vi "read Txt Files.vi"(10 "file path (use dialog)":path) -> (1 "error out":errorcluster, 2 "number":T1)   [LabVIEW 2017] (continued)
0.000000\tVoltage¡G\t-0.001160\nReal Periold(ms)¡G\t1\tEncoder Position(0.1mm)¡G\t0.000000\tVelocity(0.1mm0/s)¡G\t0.000000\tVoltage¡G\t0.000732\nReal Periold(ms)¡G\t1\tEncoder Position(0.1mm)¡G\t0.000000\tVelocity(0.1mm0/s)¡G\t0.000000\tVoltage¡G\t-0.003082\nReal Periold(ms)¡G\t1\tEncoder Position(0.1mm)¡G\t0.000000\tVelocity(0.1mm0/s)¡G\t0.000000\tVoltage¡G\t0.002319\nReal Periold(ms)¡G\t1\tEncoder Position(0.1mm)¡G\t0.000000\tVelocity(0.1mm0/s)¡G\t0.000000\tVoltage¡G\t-0.005310\nReal Periold(ms)¡G\t1\tEncoder Position(0.1mm)¡G\t0.000000\tVelocity(0.1mm0/s)¡G\t0.000000\tVoltage¡G\t-0.011688\nReal Periold(ms)¡G\t1\tEncoder Position(0.1mm)¡G\t0.000000\tVelocity(0.1mm0/s)¡G\t0.000000\tVoltage¡G\t-0.005005\nReal Periold(ms)¡G\t1\tEncoder Position(0.1mm)¡G\t0.000000\tVelocity(0.1mm0/s)¡G\t0.000000\tVoltage¡G\t0.002319\nReal Periold(ms)¡G\t1\tEncoder Position(0.1mm)¡G\t0.000000\tVelocity(0.1mm0/s)¡G\t0.000000\tVoltage¡G\t-0.006256\nReal Periold(ms)¡G\t1\tEncoder Position(0.1mm)¡G\t0.000000\tVelocity(0.1mm0/s)¡G\t0.000000\tVoltage¡G\t0.007751\nReal Periold(ms)¡G\t1\tEncoder Position(0.1mm)¡G\t0.000000\tVelocity(0.1mm0/s)¡G\t0.000000\tVoltage¡G\t0.001678\nReal Periold(ms)¡G\t1\tEncoder Position(0.1mm)¡G\t0.000000\tVelocity(0.1mm0/s)¡G\t0.000000\tVoltage¡G\t-0.000214\nReal Periold(ms)¡G\t1\tEncoder Position(0.1mm)¡G\t0.000000\tVelocity(0.1mm0/s)¡G\t0.000000\tVoltage¡G\t-0.006592\nReal Periold(ms)¡G\t1\tEncoder Position(0.1mm)¡G\t0.000000\tVelocity(0.1mm0/s)¡G\t0.000000\tVoltage¡G\t0.003296\nReal Periold(ms)¡G\t1\tEncoder Position(0.1mm)¡G\t0.000000\tVelocity(0.1mm0/s)¡G\t0.000000\tVoltage¡G\t0.005188\nReal Periold(ms)¡G\t1\tEncoder Position(0.1mm)¡G\t0.000000\tVelocity(0.1mm0/s)¡G\t0.000000\tVoltage¡G\t0.007111\nReal Periold(ms)¡G\t1\tEncoder Position(0.1mm)¡G\t0.000000\tVelocity(0.1mm0/s)¡G\t0.000000\tVoltage¡G\t-0.003387\nReal Periold(ms)¡G\t1\tEncoder Position(0.1mm)¡G\t0.000000\tVelocity(0.1mm0/s)¡G\t0.000000\tVoltage¡G\t0.001068\nReal Periold(ms)¡G\t1\tEncoder Position(0.1mm)¡G\t0.000000\tVelocity(0.1mm0/s)¡G\t0.000000\tVoltage¡G\t-0.004364\nReal Periold(ms)¡G\t1\tEncoder Position(0.1mm)¡G\t0.000000\tVelocity(0.1mm0/s)¡G\t0.000000\tVoltage¡G\t-0.001160\nReal Periold(ms)¡G\t1\tEncoder Position(0.1mm)¡G\t0.000000\tVelocity(0.1mm0/s)¡G\t0.000000\tVoltage¡G\t0.001068\nReal Periold(ms)¡G\t1\tEncoder Position(0.1mm)¡G\t0.000000\tVelocity(0.1mm0/s)¡G\t0.000000\tVoltage¡G\t0.006775\nReal Periold(ms)¡G\t1\tEncoder Position(0.1mm)¡G\t0.000000\tVelocity(0.1mm0/s)¡G\t0.000000\tVoltage¡G\t0.001373\nReal Periold(ms)¡G\t1\tEncoder Position(0.1mm)¡G\t0.000000\tVelocity(0.1mm0/s)¡G\t0.000000\tVoltage¡G\t-0.005615\nReal Periold(ms)¡G\t1\tEncoder Position(0.1mm)¡G\t0.000000\tVelocity(0.1mm0/s)¡G\t0.000000\tVoltage¡G\t-0.003723\nReal Periold(ms)¡G\t1\tEncoder Position(0.1mm)¡G\t0.000000\tVelocity(0.1mm0/s)¡G\t0.000000\tVoltage¡G\t0.003601\nReal Periold(ms)¡G\t1\tEncoder Position(0.1mm)¡G\t0.000000\tVelocity(0.1mm0/s)¡G\t0.000000\tVoltage¡G\t0.063446\nReal Periold(ms)¡G\t1\tEncoder Position(0.1mm)¡G\t0.000000\tVelocity(0.1mm0/s)¡G\t0.000000\tVoltage¡G\t-0.000214\nReal Periold(ms)¡G\t1\tEncoder Position(0.1mm)¡G\t0.000000\tVelocity(0.1mm0/s)¡G\t0.000000\tVoltage¡G\t0.006775\nReal Periold(ms)¡G\t1\tEncoder Position(0.1mm)¡G\t0.000000\tVelocity(0.1mm0/s)¡G\t0.000000\tVoltage¡G\t0.002655\nReal Periold(ms)¡G\t1\tEncoder Position(0.1mm)¡G\t0.000000\tVelocity(0.1mm0/s)¡G\t0.000000\tVoltage¡G\t-0.016754\nReal Periold(ms)¡G\t1\tEncoder Position(0.1mm)¡G\t0.000000\tVelocity(0.1mm0/s)¡G\t0.000000\tVoltage¡G\t0.001373\nReal Periold(ms)¡G\t1\tEncoder Position(0.1mm)¡G\t0.000000\tVelocity(0.1mm0/s)¡G\t0.000000\tVoltage¡G\t-0.005310\nReal Periold(ms)¡G\t1\tEncoder Position(0.1mm)¡G\t0.000000\tVelocity(0.1mm0/s)¡G\t0.000000\tVoltage¡G\t0.005188\nReal Periold(ms)¡G\t1\tEncoder Position(0.1mm)¡G\t0.000000\tVelocity(0.1mm0/s)¡G\t0.000000\tVoltage¡G\t-0.005005\nReal Periold(ms)¡G\t1\tEncoder Position(0.1mm)¡G\t0.000000\tVelocity(0.1mm0/s)¡G\t0.000000\tVoltage¡G\t0.013794\nReal Periold(ms)¡G\t1\tEncoder Position(0.1mm)¡G\t0.000000\tVelocity(0.1mm0/s)¡G\t0.000000\tVoltage¡G\t0.003906\nReal Periold(ms)¡G\t1\tEncoder Position(0.1mm)¡G\t0.000000\tVelocity(0.1mm0/s)¡G\t0.000000\tVoltage¡G\t0.052307\nReal Periold(ms)¡G\t1\tEncoder Position(0.1mm)¡G\t0.000000\tVelocity(0.1mm0/s)¡G\t0.000000\tVoltage¡G\t-0.006897\nReal Periold(ms)¡G\t1\tEncoder Position(0.1mm)¡G\t0.000000\tVelocity(0.1mm0/s)¡G\t0.000000\tVoltage¡G\t-0.028229\nReal Periold(ms)¡G\t1\tEncoder Position(0.1mm)¡G\t0.000000\tVelocity(0.1mm0/s)¡G\t0.000000\tVoltage¡G\t-0.000214\nReal Periold(ms)¡G\t1\tEncoder Position(0.1mm)¡G\t0.000000\tVelocity(0.1mm0/s)¡G\t0.000000\tVoltage¡G\t-0.008179\nReal Periold(ms)¡G\t1\tEncoder Position(0.1mm)¡G\t0.000000\tVelocity(0.1mm0/s)¡G\t0.000000\tVoltage¡G\t0.000732\nReal Periold(ms)¡G\t1\tEncoder Position(0.1mm)¡G\t0.000000\tVelocity(0.1mm0/s)¡G\t0.000000\tVoltage¡G\t-0.017395\nReal Periold(ms)¡G\t1\tEncoder Position(0.1mm)¡G\t0.000000\tVelocity(0.1mm0/s)¡G\t0.000000\tVoltage¡G\t-0.005615\nReal Periold(ms)¡G\t1\tEncoder Position(0.1mm)¡G\t0.000000\tVelocity(0.1mm0/s)¡G\t0.000000\tVoltage¡G\t-0.001495\nReal Periold(ms)¡G\t1\tEncoder Position(0.1mm)¡G\t0.000000\tVelocity(0.1mm0/s)¡G\t0.000000\tVoltage¡G\t0.001678\nReal Periold(ms)¡G\t1\tEncoder Position(0.1mm)¡G\t0.000000\tVelocity(0.1mm0/s)¡G\t0.000000\tVoltage¡G\t0.002655\nReal Periold(ms)¡G\t1\tEncoder Position(0.1mm)¡G\t0.000000\tVelocity(0.1mm0/s)¡G\t0.000000\tVoltage¡G\t0.000092\nReal Periold(ms)¡G\t1\tEncoder Position(0.1mm)¡G\t0.000000\tVelocity(0.1mm0/s)¡G\t0.000000\tVoltage¡G\t-0.046997\nReal Periold(ms)¡G\t1\tEncoder Position(0.1mm)¡G\t0.000000\tVelocity(0.1mm0/s)¡G\t0.000000\tVoltage¡G\t-0.008820\nReal Periold(ms)¡G\t1\tEncoder Position(0.1mm)¡G\t0.000000\tVelocity(0.1mm0/s)¡G\t0.000000\tVoltage¡G\t0.010284\nReal Periold(ms)¡G\t1\tEncoder Position(0.1mm)¡G\t0.000000\tVelocity(0.1mm0/s)¡G\t0.000000\tVoltage¡G\t0.009003\nReal Periold(ms)¡G\t1\tEncoder Position(0.1mm)¡G\t0.000000\tVelocity(0.1mm0/s)¡G\t0.000000\tVoltage¡G\t-0.008820\nReal Periold(ms)¡G\t1\tEncoder Position(0.1mm)¡G\t0.000000\tVelocity(0.1mm0/s)¡G\t0.000000\tVoltage¡G\t0.000427\nReal Periold(ms)¡G\t1\tEncoder Position(0.1mm)¡G\t0.000000\tVelocity(0.1mm0/s)¡G\t0.000000\tVoltage¡G\t0.001068\nReal Periold(ms)¡G\t1\tEncoder Position(0.1mm)¡G\t0.000000\tVelocity(0.1mm0/s)¡G\t0.000000\tVoltage¡G\t-0.000214\nReal Periold(ms)¡G\t1\tEncoder Position(0.1mm)¡G\t0.000000\tVelocity(0.1mm0/s)¡G\t0.000000\tVoltage¡G\t-0.003387\nReal Periold(ms)¡G\t1\tEncoder Position(0.1mm)¡G\t0.000000\tVelocity(0.1mm0/s)¡G\t0.000000\tVoltage¡G\t-0.004669\nReal Periold(ms)¡G\t1\tEncoder Position(0.1mm)¡G\t0.000000\tVelocity(0.1mm0/s)¡G\t0.000000\tVoltage¡G\t0.005188\nReal Periold(ms)¡G\t1\tEncoder Position(0.1mm)¡G\t0.000000\tVelocity(0.1mm0/s)¡G\t0.000000\tVoltage¡G\t-0.005005\nReal Periold(ms)¡G\t1\tEncoder Position(0.1mm)¡G\t0.000000\tVelocity(0.1mm0/s)¡G\t0.000000\tVoltage¡G\t0.003296\nReal Periold(ms)¡G\t1\tEncoder Position(0.1mm)¡G\t0.000000\tVelocity(0.1mm0/s)¡G\t0.000000\tVoltage¡G\t0.002655\nReal Periold(ms)¡G\t1\tEncoder Position(0.1mm)¡G\t0.000000\tVelocity(0.1mm0/s)¡G\t0.000000\tVoltage¡G\t0.001678\nReal Periold(ms)¡G\t1\tEncoder Position(0.1mm)¡G\t0.000000\tVelocity(0.1mm0/s)¡G\t0.000000\tVoltage¡G\t-0.004028\nReal Periold(ms)¡G\t1\tEncoder Position(0.1mm)¡G\t0.000000\tVelocity(0.1mm0/s)¡G\t0.000000\tVoltage¡G\t0.002960\nReal Periold(ms)¡G\t1\tEncoder Position(0.1mm)¡G\t0.000000\tVelocity(0.1mm0/s)¡G\t0.000000\tVoltage¡G\t0.018250\nReal Periold(ms)¡G\t1\tEncoder Position(0.1mm)¡G\t0.000000\tVelocity(0.1mm0/s)¡G\t0.000000\tVoltage¡G\t0.007751\nReal Periold(ms)¡G\t1\tEncoder Position(0.1mm)¡G\t0.000000\tVelocity(0.1mm0/s)¡G\t0.000000\tVoltage¡G\t0.008698\nReal Periold(ms)¡G\t1\tEncoder Position(0.1mm)¡G\t0.000000\tVelocity(0.1mm0/s)¡G\t0.000000\tVoltage¡G\t-0.002441\nReal Periold(ms)¡G\t1\tEncoder Position(0.1mm)¡G\t0.000000\tVelocity(0.1mm0/s)¡G\t0.000000\tVoltage¡G\t-0.009460\nReal Periold(ms)¡G\t1\tEncoder Position(0.1mm)¡G\t0.000000\tVelocity(0.1mm0/s)¡G\t0.000000\tVoltage¡G\t-0.005310\nReal Periold(ms)¡G\t1\tEncoder Position(0.1mm)¡G\t0.000000\tVelocity(0.1mm0/s)¡G\t0.000000\tVoltage¡G\t-0.000549\nReal Periold(ms)¡G\t1\tEncoder Position(0.1mm)¡G\t0.000000\tVelocity(0.1mm0/s)¡G\t0.000000\tVoltage¡G\t0.002319\nReal Periold(ms)¡G\t1\tEncoder Position(0.1mm)¡G\t0.000000\tVelocity(0.1mm0/s)¡G\t0.000000\tVoltage¡G\t-0.014526\nReal Periold(ms)¡G\t1\tEncoder Position(0.1mm)¡G\t0.000000\tVelocity(0.1mm0/s)¡G\t0.000000\tVoltage¡G\t-0.012939\nReal Periold(ms)¡G\t1\tEncoder Position(0.1mm)¡G\t0.000000\tVelocity(0.1mm0/s)¡G\t0.000000\tVoltage¡G\t0.006470\nReal Periold(ms)¡G\t1\tEncoder Position(0.1mm)¡G\t0.000000\tVelocity(0.1mm0/s)¡G\t0.000000\tVoltage¡G\t0.001068\nReal Periold(ms)¡G\t1\tEncoder Position(0.1mm)¡G\t0.000000\tVelocity(0.1mm0/s)¡G\t0.000000\tVoltage¡G\t-0.003387\nReal Periold(ms)¡G\t1\tEncoder Position(0.1mm)¡G\t0.000000\tVelocity(0.1mm0/s)¡G\t0.000000\tVoltage¡G\t0.008057\nReal Periold(ms)¡G\t1\tEncoder Position(0.1mm)¡G\t0.000000\tVelocity(0.1mm0/s)¡G\t0.000000\tVoltage¡G\t-0.001801\nReal Periold(ms)¡G\t1\tEncoder Position(0.1mm)¡G\t0.000000\tVelocity(0.1mm0/s)¡G\t0.000000\tVoltage¡G\t0.003296\nReal Periold(ms)¡G\t1\tEncoder Position(0.1mm)¡G\t0.000000\tVelocity(0.1mm0/s)¡G\t0.000000\tVoltage¡G\t-0.007538\nReal Periold(ms)¡G\t1\tEncoder Position(0.1mm)¡G\t0.000000\tVelocity(0.1mm0/s)¡G\t0.000000\tVoltage¡G\t-0.010712\nReal Periold(ms)¡G\t1\tEncoder Position(0.1mm)¡G\t0.000000\tVelocity(0.1mm0/s)¡G\t0.000000\tVoltage¡G\t-0.007843\nReal Periold(ms)¡G\t1\tEncoder Position(0.1mm)¡G\t0.000000\tVelocity(0.1mm0/s)¡G\t0.000000\tVoltage¡G\t-0.001160\nReal Periold(ms)¡G\t1\tEncoder Position(0.1mm)¡G\t0.000000\tVelocity(0.1mm0/s)¡G\t0.000000\tVoltage¡G\t0.003296\nReal Periold(ms)¡G\t1\tEncoder Position(0.1mm)¡G\t0.000000\tVelocity(0.1mm0/s)¡G\t0.000000\tVoltage¡G\t0.001373\nReal Periold(ms)¡G\t1\tEncoder Position(0.1mm)¡G\t0.000000\tVelocity(0.1mm0/s)¡G\t0.000000\tVoltage¡G\t-0.016144\nReal Periold(ms)¡G\t1\tEncoder Position(0.1mm)¡G\t0.000000\tVelocity(0.1mm0/s)¡G\t0.000000\tVoltage¡G\t0.000427\nReal Periold(ms)¡G\t1\tEncoder Position(0.1mm)¡G\t0.000000\tVelocity(0.1mm0/s)¡G\t0.000000\tVoltage¡G\t-0.010406\nReal Periold(ms)¡G\t1\tEncoder Position(0.1mm)¡G\t0.000000\tVelocity(0.1mm0/s)¡G\t0.000000\tVoltage¡G\t0.006134\nReal Periold(ms)¡G\t1\tEncoder Position(0.1mm)¡G\t0.000000\tVelocity(0.1mm0/s)¡G\t0.000000\tVoltage¡G\t0.003296\nReal Periold(ms)¡G\t1\tEncoder Position(0.1mm)¡G\t0.000000\tVelocity(0.1mm0/s)¡G\t0.000000\tVoltage¡G\t0.004547\nReal Periold(ms)¡G\t1\tEncoder Position(0.1mm)¡G\t0.000000\tVelocity(0.1mm0/s)¡G\t0.000000\tVoltage¡G\t-0.008179\nReal Periold(ms)¡G\t1\tEncoder Position(0.1mm)¡G\t0.000000\tVelocity(0.1mm0/s)¡G\t0.000000\tVoltage¡G\t-0.005005\nReal Periold(ms)¡G\t1\tEncoder Position(0.1mm)¡G\t0.000000\tVelocity(0.1mm0/s)¡G\t0.000000\tVoltage¡G\t0.011566\nReal Periold(ms)¡G\t1\tEncoder Position(0.1mm)¡G\t0.000000\tVelocity(0.1mm0/s)¡G\t0.000000\tVoltage¡G\t0.001068\nReal Periold(ms)¡G\t1\tEncoder Position(0.1mm)¡G\t0.000000\tVelocity(0.1mm0/s)¡G\t0.000000\tVoltage¡G\t-0.002136\nReal Periold(ms)¡G\t1\tEncoder Position(0.1mm)¡G\t0.000000\tVelocity(0.1mm0/s)¡G\t0.000000\tVoltage¡G\t-0.005615\nReal Periold(ms)¡G\t1\tEncoder Position(0.1mm)¡G\t0.000000\tVelocity(0.1mm0/s)¡G\t0.000000\tVoltage¡G\t-0.003723\nReal Periold(ms)¡G\t1\tEncoder Position(0.1mm)¡G\t0.000000\tVelocity(0.1mm0/s)¡G\t0.000000\tVoltage¡G\t0.001678\nReal Periold(ms)¡G\t1\tEncoder Position(0.1mm)¡G\t0.000000\tVelocity(0.1mm0/s)¡G\t0.000000\tVoltage¡G\t-0.005615\nReal Periold(ms)¡G\t1\tEncoder Position(0.1mm)¡G\t0.000000\tVelocity(0.1mm0/s)¡G\t0.000000\tVoltage¡G\t0.009338\nReal Periold(ms)¡G\t1\tEncoder Position(0.1mm)¡G\t0.000000\tVelocity(0.1mm0/s)¡G\t0.000000\tVoltage¡G\t0.007416\nReal Periold(ms)¡G\t1\tEncoder Position(0.1mm)¡G\t0.000000\tVelocity(0.1mm0/s)¡G\t0.000000\tVoltage¡G\t0.038940\nReal Periold(ms)¡G\t1\tEncoder Position(0.1mm)¡G\t0.000000\tVelocity(0.1mm0/s)¡G\t0.000000\tVoltage¡G\t-0.007233\nReal Periold(ms)¡G\t1\tEncoder Position(0.1mm)¡G\t0.000000\tVelocity(0.1mm0/s)¡G\t0.000000\tVoltage¡G\t0.000092\nReal Periold(ms)¡G\t1\tEncoder Position(0.1mm)¡G\t0.000000\tVelocity(0.1mm0/s)¡G\t0.000000\tVoltage¡G\t-0.001495\nReal Periold(ms)¡G\t1\tEncoder Position(0.1mm)¡G\t0.000000\tVelocity(0.1mm0/s)¡G\t0.000000\tVoltage¡G\t-0.006592\nReal Periold(ms)¡G\t1\tEncoder Position(0.1mm)¡G\t0.000000\tVelocity(0.1mm0/s)¡G\t0.000000\tVoltage¡G\t0.049744\nReal Periold(ms)¡G\t1\tEncoder Position(0.1mm)¡G\t0.000000\tVelocity(0.1mm0/s)¡G\t0.000000\tVoltage¡G\t-0.012299\nReal Periold(ms)¡G\t1\tEncoder Position(0.1mm)¡G\t0.000000\tVelocity(0.1mm0/s)¡G\t0.000000\tVoltage¡G\t-0.004028\nReal Periold(ms)¡G\t1\tEncoder Position(0.1mm)¡G\t0.000000\tVelocity(0.1mm0/s)¡G\t0.000000\tVoltage¡G\t0.059631\nReal Periold(ms)¡G\t1\tEncoder Position(0.1mm)¡G\t0.000000\tVelocity(0.1mm0/s)¡G\t0.000000\tVoltage¡G\t0.005829\nReal Periold(ms)¡G\t1\tEncoder Position(0.1mm)¡G\t0.000000\tVelocity(0.1mm0/s)¡G\t0.000000\tVoltage¡G\t-0.009125\nReal Periold(ms)¡G\t1\tEncoder Position(0.1mm)¡G\t0.000000\tVelocity(0.1mm0/s)¡G\t0.000000\tVoltage¡G\t0.023346\nReal Periold(ms)¡G\t1\tEncoder Position(0.1mm)¡G\t0.000000\tVelocity(0.1mm0/s)¡G\t0.000000\tVoltage¡G\t-0.008179\nReal Periold(ms)¡G\t1\tEncoder Position(0.1mm)¡G\t0.000000\tVelocity(0.1mm0/s)¡G\t0.000000\tVoltage¡G\t-0.007538\nReal Periold(ms)¡G\t1\tEncoder Position(0.1mm)¡G\t0.000000\tVelocity(0.1mm0/s)¡G\t0.000000\tVoltage¡G\t-0.011993\nReal Periold(ms)¡G\t1\tEncoder Position(0.1mm)¡G\t0.000000\tVelocity(0.1mm0/s)¡G\t0.000000\tVoltage¡G\t-0.000214\nReal Periold(ms)¡G\t1\tEncoder Position(0.1mm)¡G\t0.000000\tVelocity(0.1mm0/s)¡G\t0.000000\tVoltage¡G\t-0.000854\nReal Periold(ms)¡G\t1\tEncoder Position(0.1mm)¡G\t0.000000\tVelocity(0.1mm0/s)¡G\t0.000000\tVoltage¡G\t-0.006592\nReal Periold(ms)¡G\t1\tEncoder Position(0.1mm)¡G\t0.000000\tVelocity(0.1mm0/s)¡G\t0.000000\tVoltage¡G\t-0.003723\nReal Periold(ms)¡G\t1\tEncoder Position(0.1mm)¡G\t0.000000\tVelocity(0.1mm0/s)¡G\t0.000000\tVoltage¡G\t0.000732\nReal Periold(ms)¡G\t1\tEncoder Position(0.1mm)¡G\t0.000000\tVelocity(0.1mm0/s)¡G\t0.000000\tVoltage¡G\t0.001373\nReal Periold(ms)¡G\t1\tEncoder Position(0.1mm)¡G\t0.000000\tVelocity(0.1mm0/s)¡G\t0.000000\tVoltage¡G\t-0.005951\nReal Periold(ms)¡G\t1\tEncoder Position(0.1mm)¡G\t0.000000\tVelocity(0.1mm0/s)¡G\t0.000000\tVoltage¡G\t0.002014\nReal Periold(ms)¡G\t1\tEncoder Position(0.1mm)¡G\t0.000000\tVelocity(0.1mm0/s)¡G\t0.000000\tVoltage¡G\t0.011230\nReal Periold(ms)¡G\t1\tEncoder Position(0.1mm)¡G\t0.000000\tVelocity(0.1mm0/s)¡G\t0.000000\tVoltage¡G\t-0.010406\nReal Periold(ms)¡G\t1\tEncoder Position(0.1mm)¡G\t0.000000\tVelocity(0.1mm0/s)¡G\t0.000000\tVoltage¡G\t0.002319\nReal Periold(ms)¡G\t1\tEncoder Position(0.1mm)¡G\t0.000000\tVelocity(0.1mm0/s)¡G\t0.000000\tVoltage¡G\t-0.000549\nReal Periold(ms)¡G\t1\tEncoder Position(0.1mm)¡G\t0.000000\tVelocity(0.1mm0/s)¡G\t0.000000\tVoltage¡G\t0.003601\nReal Periold(ms)¡G\t1\tEncoder Position(0.1mm)¡G\t0.000000\tVelocity(0.1mm0/s)¡G\t0.000000\tVoltage¡G\t-0.000854\nReal Periold(ms)¡G\t1\tEncoder Position(0.1mm)¡G\t0.000000\tVelocity(0.1mm0/s)¡G\t0.000000\tVoltage¡G\t-0.010406\nReal Periold(ms)¡G\t1\tEncoder Position(0.1mm)¡G\t0.000000\tVelocity(0.1mm0/s)¡G\t0.000000\tVoltage¡G\t-0.003387\nReal Periold(ms)¡G\t1\tEncoder Position(0.1mm)¡G\t0.000000\tVelocity(0.1mm0/s)¡G\t0.000000\tVoltage¡G\t-0.001495\nReal Periold(ms)¡G\t1\tEncoder Position(0.1mm)¡G\t0.000000\tVelocity(0.1mm0/s)¡G\t0.000000\tVoltage¡G\t-0.006256\nReal Periold(ms)¡G\t1\tEncoder Position(0.1mm)¡G\t0.000000\tVelocity(0.1mm0/s)¡G\t0.000000\tVoltage¡G\t0.006134\nReal Periold(ms)¡G\t1\tEncoder Position(0.1mm)¡G\t0.000000\tVelocity(0.1mm0/s)¡G\t0.000000\tVoltage¡G\t-0.005951\nReal Periold(ms)¡G\t1\tEncoder Position(0.1mm)¡G\t0.000000\tVelocity(0.1mm0/s)¡G\t0.000000\tVoltage¡G\t-0.002136\nReal Periold(ms)¡G\t1\tEncoder Position(0.1mm)¡G\t0.000000\tVelocity(0.1mm0/s)¡G\t0.000000\tVoltage¡G\t0.006470\nReal Periold(ms)¡G\t1\tEncoder Position(0.1mm)¡G\t0.000000\tVelocity(0.1mm0/s)¡G\t0.000000\tVoltage¡G\t-0.000214\nReal Periold(ms)¡G\t1\tEncoder Position(0.1mm)¡G\t0.000000\tVelocity(0.1mm0/s)¡G\t0.000000\tVoltage¡G\t0.002014\nReal Periold(ms)¡G\t1\tEncoder Position(0.1mm)¡G\t0.000000\tVelocity(0.1mm0/s)¡G\t0.000000\tVoltage¡G\t0.004883\nReal Periold(ms)¡G\t1\tEncoder Position(0.1mm)¡G\t0.000000\tVelocity(0.1mm0/s)¡G\t0.000000\tVoltage¡G\t-0.003082\nReal Periold(ms)¡G\t1\tEncoder Position(0.1mm)¡G\t0.000000\tVelocity(0.1mm0/s)¡G\t0.000000\tVoltage¡G\t-0.001495\nReal Periold(ms)¡G\t1\tEncoder Position(0.1mm)¡G\t0.000000\tVelocity(0.1mm0/s)¡G\t0.000000\tVoltage¡G\t0.000092\nReal Periold(ms)¡G\t1\tEncoder Position(0.1mm)¡G\t0.000000\tVelocity(0.1mm0/s)¡G\t0.000000\tVoltage¡G\t-0.005005\nReal Periold(ms)¡G\t1\tEncoder Position(0.1mm)¡G\t0.000000\tVelocity(0.1mm0/s)¡G\t0.000000\tVoltage¡G\t0.001678\nReal Periold(ms)¡G\t1\tEncoder Position(0.1mm)¡G\t0.000000\tVelocity(0.1mm0/s)¡G\t0.000000\tVoltage¡G\t-0.013580\nReal Periold(ms)¡G\t1\tEncoder Position(0.1mm)¡G\t0.000000\tVelocity(0.1mm0/s)¡G\t0.000000\tVoltage¡G\t0.013794\nReal Periold(ms)¡G\t1\tEncoder Position(0.1mm)¡G\t0.000000\tVelocity(0.1mm0/s)¡G\t0.000000\tVoltage¡G\t0.012207\nReal Periold(ms)¡G\t1\tEncoder Position(0.1mm)¡G\t0.000000\tVelocity(0.1mm0/s)¡G\t0.000000\tVoltage¡G\t0.005829\nReal Periold(ms)¡G\t1\tEncoder Position(0.1mm)¡G\t0.000000\tVelocity(0.1mm0/s)¡G\t0.000000\tVoltage¡G\t-0.005951\nReal Periold(ms)¡G\t1\tEncoder Position(0.1mm)¡G\t0.000000\tVelocity(0.1mm0/s)¡G\t0.000000\tVoltage¡G\t-0.004028\nReal Periold(ms)¡G\t1\tEncoder Position(0.1mm)¡G\t0.000000\tVelocity(0.1mm0/s)¡G\t0.000000\tVoltage¡G\t0.002014\nReal Periold(ms)¡G\t1\tEncoder Position(0.1mm)¡G\t0.000000\tVelocity(0.1mm0/s)¡G\t0.000000\tVoltage¡G\t0.004883\nReal Periold(ms)¡G\t1\tEncoder Position(0.1mm)¡G\t0.000000\tVelocity(0.1mm0/s)¡G\t0.000000\tVoltage¡G\t-0.006256\nReal Periold(ms)¡G\t1\tEncoder Position(0.1mm)¡G\t0.000000\tVelocity(0.1mm0/s)¡G\t0.000000\tVoltage¡G\t-0.010071\nReal Periold(ms)¡G\t1\tEncoder Position(0.1mm)¡G\t0.000000\tVelocity(0.1mm0/s)¡G\t0.000000\tVoltage¡G\t-0.002777\nReal Periold(ms)¡G\t1\tEncoder Position(0.1mm)¡G\t0.000000\tVelocity(0.1mm0/s)¡G\t0.000000\tVoltage¡G\t0.003296\nReal Periold(ms)¡G\t1\tEncoder Position(0.1mm)¡G\t0.000000\tVelocity(0.1mm0/s)¡G\t0.000000\tVoltage¡G\t-0.005310\nReal Periold(ms)¡G\t1\tEncoder Position(0.1mm)¡G\t0.000000\tVelocity(0.1mm0/s)¡G\t0.000000\tVoltage¡G\t-0.005951\nReal Periold(ms)¡G\t1\tEncoder Position(0.1mm)¡G\t0.000000\tVelocity(0.1mm0/s)¡G\t0.000000\tVoltage¡G\t-0.011688\nReal Periold(ms)¡G\t1\tEncoder Position(0.1mm)¡G\t0.000000\tVelocity(0.1mm0/s)¡G\t0.000000\tVoltage¡G\t-0.017395\nReal Periold(ms)¡G\t1\tEncoder Position(0.1mm)¡G\t0.000000\tVelocity(0.1mm0/s)¡G\t0.000000\tVoltage¡G\t0.011230\nReal Periold(ms)¡G\t1\tEncoder Position(0.1mm)¡G\t0.000000\tVelocity(0.1mm0/s)¡G\t0.000000\tVoltage¡G\t0.017609\nReal Periold(ms)¡G\t1\tEncoder Position(0.1mm)¡G\t0.000000\tVelocity(0.1mm0/s)¡G\t0.000000\tVoltage¡G\t-0.001801\nReal Periold(ms)¡G\t1\tEncoder Position(0.1mm)¡G\t0.000000\tVelocity(0.1mm0/s)¡G\t0.000000\tVoltage¡G\t-0.022491\nReal Periold(ms)¡G\t1\tEncoder Position(0.1mm)¡G\t0.000000\tVelocity(0.1mm0/s)¡G\t0.000000\tVoltage¡G\t-0.007538\nReal Periold(ms)¡G\t1\tEncoder Position(0.1mm)¡G\t0.000000\tVelocity(0.1mm0/s)¡G\t0.000000\tVoltage¡G\t0.006134\nReal Periold(ms)¡G\t1\tEncoder Position(0.1mm)¡G\t0.000000\tVelocity(0.1mm0/s)¡G\t0.000000\tVoltage¡G\t-0.015808\nReal Periold(ms)¡G\t1\tEncoder Position(0.1mm)¡G\t0.000000\tVelocity(0.1mm0/s)¡G\t0.000000\tVoltage¡G\t0.002014\nReal Periold(ms)¡G\t1\tEncoder Position(0.1mm)¡G\t0.000000\tVelocity(0.1mm0/s)¡G\t0.000000\tVoltage¡G\t-0.005615\nReal Periold(ms)¡G\t1\tEncoder Position(0.1mm)¡G\t0.000000\tVelocity(0.1mm0/s)¡G\t0.000000\tVoltage¡G\t-0.006897\nReal Periold(ms)¡G\t1\tEncoder Position(0.1mm)¡G\t0.000000\tVelocity(0.1mm0/s)¡G\t0.000000\tVoltage¡G\t-0.001495\nReal Periold(ms)¡G\t1\tEncoder Position(0.1mm)¡G\t0.000000\tVelocity(0.1mm0/s)¡G\t0.000000\tVoltage¡G\t0.005524\nReal Periold(ms)¡G\t1\tEncoder Position(0.1mm)¡G\t0.000000\tVelocity(0.1mm0/s)¡G\t0.000000\tVoltage¡G\t0.002960\nReal Periold(ms)¡G\t1\tEncoder Position(0.1mm)¡G\t0.000000\tVelocity(0.1mm0/s)¡G\t0.000000\tVoltage¡G\t-0.002777\nReal Periold(ms)¡G\t1\tEncoder Position(0.1mm)¡G\t0.000000\tVelocity(0.1mm0/s)¡G\t0.000000\tVoltage¡G\t0.000092\nReal Periold(ms)¡G\t1\tEncoder Position(0.1mm)¡G\t0.000000\tVelocity(0.1mm0/s)¡G\t0.000000\tVoltage¡G\t-0.019318\nReal Periold(ms)¡G\t1\tEncoder Position(0.1mm)¡G\t0.000000\tVelocity(0.1mm0/s)¡G\t0.000000\tVoltage¡G\t0.000732\nReal Periold(ms)¡G\t1\tEncoder Position(0.1mm)¡G\t0.000000\tVelocity(0.1mm0/s)¡G\t0.000000\tVoltage¡G\t-0.005310\nReal Periold(ms)¡G\t1\tEncoder Position(0.1mm)¡G\t0.000000\tVelocity(0.1mm0/s)¡G\t0.000000\tVoltage¡G\t0.006134\nReal Periold(ms)¡G\t1\tEncoder Position(0.1mm)¡G\t0.000000\tVelocity(0.1mm0/s)¡G\t0.000000\tVoltage¡G\t-0.003723\nReal Periold(ms)¡G\t1\tEncoder Position(0.1mm)¡G\t0.000000\tVelocity(0.1mm0/s)¡G\t0.000000\tVoltage¡G\t-0.008820\nReal Periold(ms)¡G\t1\tEncoder Position(0.1mm)¡G\t0.000000\tVelocity(0.1mm0/s)¡G\t0.000000\tVoltage¡G\t-0.003082\nReal Periold(ms)¡G\t1\tEncoder Position(0.1mm)¡G\t0.000000\tVelocity(0.1mm0/s)¡G\t0.000000\tVoltage¡G\t0.010590\nReal Periold(ms)¡G\t1\tEncoder Position(0.1mm)¡G\t0.000000\tVelocity(0.1mm0/s)¡G\t0.000000\tVoltage¡G\t-0.005005\nReal Periold(ms)¡G\t1\tEncoder Position(0.1mm)¡G\t0.000000\tVelocity(0.1mm0/s)¡G\t0.000000\tVoltage¡G\t-0.002136\nReal Periold(ms)¡G\t1\tEncoder Position(0.1mm)¡G\t0.000000\tVelocity(0.1mm0/s)¡G\t0.000000\tVoltage¡G\t-0.000214\nReal Periold(ms)¡G\t1\tEncoder Position(0.1mm)¡G\t0.000000\tVelocity(0.1mm0/s)¡G\t0.000000\tVoltage¡G\t-0.003082\nReal Periold(ms)¡G\t1\tEncoder Position(0.1mm)¡G\t0.000000\tVelocity(0.1mm0/s)¡G\t0.000000\tVoltage¡G\t-0.002136\nReal Periold(ms)¡G\t1\tEncoder Position(0.1mm)¡G\t0.000000\tVelocity(0.1mm0/s)¡G\t0.000000\tVoltage¡G\t-0.005615\nReal Periold(ms)¡G\t1\tEncoder Position(0.1mm)¡G\t0.000000\tVelocity(0.1mm0/s)¡G\t0.000000\tVoltage¡G\t-0.007233\nReal Periold(ms)¡G\t1\tEncoder Position(0.1mm)¡G\t0.000000\tVelocity(0.1mm0/s)¡G\t0.000000\tVoltage¡G\t-0.021240\nReal Periold(ms)¡G\t1\tEncoder Position(0.1mm)¡G\t0.000000\tVelocity(0.1mm0/s)¡G\t0.000000\tVoltage¡G\t-0.006256\nReal Periold(ms)¡G\t1\tEncoder Position(0.1mm)¡G\t0.000000\tVelocity(0.1mm0/s)¡G\t0.000000\tVoltage¡G\t-0.006897\nReal Periold(ms)¡G\t1\tEncoder Position(0.1mm)¡G\t0.000000\tVelocity(0.1mm0/s)¡G\t0.000000\tVoltage¡G\t-0.000549\nReal Periold(ms)¡G\t1\tEncoder Position(0.1mm)¡G\t0.000000\tVelocity(0.1mm0/s)¡G\t0.000000\tVoltage¡G\t-0.002441\nReal Periold(ms)¡G\t1\tEncoder Position(0.1mm)¡G\t0.000000\tVelocity(0.1mm0/s)¡G\t0.000000\tVoltage¡G\t-0.000214\nReal Periold(ms)¡G\t1\tEncoder Position(0.1mm)¡G\t0.000000\tVelocity(0.1mm0/s)¡G\t0.000000\tVoltage¡G\t0.000732\nReal Periold(ms)¡G\t1\tEncoder Position(0.1mm)¡G\t0.000000\tVelocity(0.1mm0/s)¡G\t0.000000\tVoltage¡G\t-0.018982\nReal Periold(ms)¡G\t1\tEncoder Position(0.1mm)¡G\t0.000000\tVelocity(0.1mm0/s)¡G\t0.000000\tVoltage¡G\t0.010590\nReal Periold(ms)¡G\t1\tEncoder Position(0.1mm)¡G\t0.000000\tVelocity(0.1mm0/s)¡G\t0.000000\tVoltage¡G\t-0.008484\nReal Periold(ms)¡G\t1\tEncoder Position(0.1mm)¡G\t0.000000\tVelocity(0.1mm0/s)¡G\t0.000000\tVoltage¡G\t-0.013916\nReal Periold(ms)¡G\t1\tEncoder Position(0.1mm)¡G\t0.000000\tVelocity(0.1mm0/s)¡G\t0.000000\tVoltage¡G\t0.001373\nReal Periold(ms)¡G\t1\tEncoder Position(0.1mm)¡G\t0.000000\tVelocity(0.1mm0/s)¡G\t0.000000\tVoltage¡G\t-0.008820\nReal Periold(ms)¡G\t1\tEncoder Position(0.1mm)¡G\t0.000000\tVelocity(0.1mm0/s)¡G\t0.000000\tVoltage¡G\t-0.001495\nReal Periold(ms)¡G\t1\tEncoder Position(0.1mm)¡G\t0.000000\tVelocity(0.1mm0/s)¡G\t0.000000\tVoltage¡G\t0.005188\nReal Periold(ms)¡G\t1\tEncoder Position(0.1mm)¡G\t0.000000\tVelocity(0.1mm0/s)¡G\t0.000000\tVoltage¡G\t0.003906\nReal Periold(ms)¡G\t1\tEncoder Position(0.1mm)¡G\t0.000000\tVelocity(0.1mm0/s)¡G\t0.000000\tVoltage¡G\t0.016022\nReal Periold(ms)¡G\t1\tEncoder Position(0.1mm)¡G\t0.000000\tVelocity(0.1mm0/s)¡G\t0.000000\tVoltage¡G\t-0.006256\nReal Periold(ms)¡G\t1\tEncoder Position(0.1mm)¡G\t0.000000\tVelocity(0.1mm0/s)¡G\t0.000000\tVoltage¡G\t0.002655\nReal Periold(ms)¡G\t1\tEncoder Position(0.1mm)¡G\t0.000000\tVelocity(0.1mm0/s)¡G\t0.000000\tVoltage¡G\t-0.003387\nReal Periold(ms)¡G\t1\tEncoder Position(0.1mm)¡G\t0.000000\tVelocity(0.1mm0/s)¡G\t0.000000\tVoltage¡G\t-0.003387\nReal Periold(ms)¡G\t1\tEncoder Position(0.1mm)¡G\t0.000000\tVelocity(0.1mm0/s)¡G\t0.000000\tVoltage¡G\t-0.007538\nReal Periold(ms)¡G\t1\tEncoder Position(0.1mm)¡G\t0.000000\tVelocity(0.1mm0/s)¡G\t0.000000\tVoltage¡G\t0.011566\nReal Periold(ms)¡G\t1\tEncoder Position(0.1mm)¡G\t0.000000\tVelocity(0.1mm0/s)¡G\t0.000000\tVoltage¡G\t0.014099\nReal Periold(ms)¡G\t1\tEncoder Position(0.1mm)¡G\t0.000000\tVelocity(0.1mm0/s)¡G\t0.000000\tVoltage¡G\t-0.000854\nReal Periold(ms)¡G\t1\tEncoder Position(0.1mm)¡G\t0.000000\tVelocity(0.1mm0/s)¡G\t0.000000\tVoltage¡G\t0.000092\nReal Periold(ms)¡G\t1\tEncoder Position(0.1mm)¡G\t0.000000\tVelocity(0.1mm0/s)¡G\t0.000000\tVoltage¡G\t-0.002441\nReal Periold(ms)¡G\t1\tEncoder Position(0.1mm)¡G\t0.000000\tVelocity(0.1mm0/s)¡G\t0.000000\tVoltage¡G\t-0.002441\nReal Periold(ms)¡G\t1\tEncoder Position(0.1mm)¡G\t0.000000\tVelocity(0.1mm0/s)¡G\t0.000000\tVoltage¡G\t-0.008820\nReal Periold(ms)¡G\t1\tEncoder Position(0.1mm)¡G\t0.000000\tVelocity(0.1mm0/s)¡G\t0.000000\tVoltage¡G\t-0.004028\nReal Periold(ms)¡G\t1\tEncoder Position(0.1mm)¡G\t0.000000\tVelocity(0.1mm0/s)¡G\t0.000000\tVoltage¡G\t-0.011993\nReal Periold(ms)¡G\t1\tEncoder Position(0.1mm)¡G\t0.000000\tVelocity(0.1mm0/s)¡G\t0.000000\tVoltage¡G\t-0.015808\nReal Periold(ms)¡G\t1\tEncoder Position(0.1mm)¡G\t0.000000\tVelocity(0.1mm0/s)¡G\t0.000000\tVoltage¡G\t0.005524\nReal Periold(ms)¡G\t1\tEncoder Position(0.1mm)¡G\t0.000000\tVelocity(0.1mm0/s)¡G\t0.000000\tVoltage¡G\t-0.005005\nReal Periold(ms)¡G\t1\tEncoder Position(0.1mm)¡G\t0.000000\tVelocity(0.1mm0/s)¡G\t0.000000\tVoltage¡G\t-0.004364\nReal Periold(ms)¡G\t1\tEncoder Position(0.1mm)¡G\t0.000000\tVelocity(0.1mm0/s)¡G\t0.000000\tVoltage¡G\t0.003906\nReal Periold(ms)¡G\t1\tEncoder Position(0.1mm)¡G\t0.000000\tVelocity(0.1mm0/s)¡G\t0.000000\tVoltage¡G\t-0.000214\nReal Periold(ms)¡G\t1\tEncoder Position(0.1mm)¡G\t0.000000\tVelocity(0.1mm0/s)¡G\t0.000000\tVoltage¡G\t-0.007233\nReal Periold(ms)¡G\t1\tEncoder Position(0.1mm)¡G\t0.000000\tVelocity(0.1mm0/s)¡G\t0.000000\tVoltage¡G\t-0.005951\nReal Periold(ms)¡G\t1\tEncoder Position(0.1mm)¡G\t0.000000\tVelocity(0.1mm0/s)¡G\t0.000000\tVoltage¡G\t-0.001495\nReal Periold(ms)¡G\t1\tEncoder Position(0.1mm)¡G\t0.000000\tVelocity(0.1mm0/s)¡G\t0.000000\tVoltage¡G\t-0.016754\nReal Periold(ms)¡G\t1\tEncoder Position(0.1mm)¡G\t0.000000\tVelocity(0.1mm0/s)¡G\t0.000000\tVoltage¡G\t-0.002777\nReal Periold(ms)¡G\t1\tEncoder Position(0.1mm)¡G\t0.000000\tVelocity(0.1mm0/s)¡G\t0.000000\tVoltage¡G\t0.005524\nReal Periold(ms)¡G\t1\tEncoder Position(0.1mm)¡G\t0.000000\tVelocity(0.1mm0/s)¡G\t0.000000\tVoltage¡G\t-0.001160\nReal Periold(ms)¡G\t1\tEncoder Position(0.1mm)¡G\t0.000000\tVelocity(0.1mm0/s)¡G\t0.000000\tVoltage¡G\t-0.008484\nReal Periold(ms)¡G\t1\tEncoder Position(0.1mm)¡G\t0.000000\tVelocity(0.1mm0/s)¡G\t0.000000\tVoltage¡G\t-0.001495\nReal Periold(ms)¡G\t1\tEncoder Position(0.1mm)¡G\t0.000000\tVelocity(0.1mm0/s)¡G\t0.000000\tVoltage¡G\t0.003906\nReal Periold(ms)¡G\t1\tEncoder Position(0.1mm)¡G\t0.000000\tVelocity(0.1mm0/s)¡G\t0.000000\tVoltage¡G\t0.016022\nReal Periold(ms)¡G\t1\tEncoder Position(0.1mm)¡G\t0.000000\tVelocity(0.1mm0/s)¡G\t0.000000\tVoltage¡G\t0.008362\nReal Periold(ms)¡G\t1\tEncoder Position(0.1mm)¡G\t0.000000\tVelocity(0.1mm0/s)¡G\t0.000000\tVoltage¡G\t-0.027283\nReal Periold(ms)¡G\t1\tEncoder Position(0.1mm)¡G\t0.000000\tVelocity(0.1mm0/s)¡G\t0.000000\tVoltage¡G\t-0.014526\nReal Periold(ms)¡G\t1\tEncoder Position(0.1mm)¡G\t0.000000\tVelocity(0.1mm0/s)¡G\t0.000000\tVoltage¡G\t-0.001495\nReal Periold(ms)¡G\t1\tEncoder Position(0.1mm)¡G\t0.000000\tVelocity(0.1mm0/s)¡G\t0.000000\tVoltage¡G\t-0.011993\nReal Periold(ms)¡G\t1\tEncoder Position(0.1mm)¡G\t0.000000\tVelocity(0.1mm0/s)¡G\t0.000000\tVoltage¡G\t0.003906\nReal Periold(ms)¡G\t1\tEncoder Position(0.1mm)¡G\t0.000000\tVelocity(0.1mm0/s)¡G\t0.000000\tVoltage¡G\t0.003601\nReal Periold(ms)¡G\t1\tEncoder Position(0.1mm)¡G\t0.000000\tVelocity(0.1mm0/s)¡G\t0.000000\tVoltage¡G\t0.000732\nReal Periold(ms)¡G\t1\tEncoder Position(0.1mm)¡G\t0.000000\tVelocity(0.1mm0/s)¡G\t0.000000\tVoltage¡G\t-0.004364\nReal Periold(ms)¡G\t1\tEncoder Position(0.1mm)¡G\t0.000000\tVelocity(0.1mm0/s)¡G\t0.000000\tVoltage¡G\t0.001373\nReal Periold(ms)¡G\t1\tEncoder Position(0.1mm)¡G\t0.000000\tVelocity(0.1mm0/s)¡G\t0.000000\tVoltage¡G\t0.003906\nReal Periold(ms)¡G\t1\tEncoder Position(0.1mm)¡G\t0.000000\tVelocity(0.1mm0/s)¡G\t0.000000\tVoltage¡G\t-0.005951\nReal Periold(ms)¡G\t1\tEncoder Position(0.1mm)¡G\t0.000000\tVelocity(0.1mm0/s)¡G\t0.000000\tVoltage¡G\t-0.005005\nReal Periold(ms)¡G\t1\tEncoder Position(0.1mm)¡G\t0.000000\tVelocity(0.1mm0/s)¡G\t0.000000\tVoltage¡G\t-0.007843\nReal Periold(ms)¡G\t1\tEncoder Position(0.1mm)¡G\t0.000000\tVelocity(0.1mm0/s)¡G\t0.000000\tVoltage¡G\t0.011230\nReal Periold(ms)¡G\t1\tEncoder Position(0.1mm)¡G\t0.000000\tVelocity(0.1mm0/s)¡G\t0.000000\tVoltage¡G\t0.001678\nReal Periold(ms)¡G\t1\tEncoder Position(0.1mm)¡G\t0.000000\tVelocity(0.1mm0/s)¡G\t0.000000\tVoltage¡G\t0.004242\nReal Periold(ms)¡G\t1\tEncoder Position(0.1mm)¡G\t0.000000\tVelocity(0.1mm0/s)¡G\t0.000000\tVoltage¡G\t0.016663\nReal Periold(ms)¡G\t1\tEncoder Position(0.1mm)¡G\t0.000000\tVelocity(0.1mm0/s)¡G\t0.000000\tVoltage¡G\t-0.001801\nReal Periold(ms)¡G\t1\tEncoder Position(0.1mm)¡G\t0.000000\tVelocity(0.1mm0/s)¡G\t0.000000\tVoltage¡G\t-0.001495\nReal Periold(ms)¡G\t1\tEncoder Position(0.1mm)¡G\t0.000000\tVelocity(0.1mm0/s)¡G\t0.000000\tVoltage¡G\t0.005829\nReal Periold(ms)¡G\t1\tEncoder Position(0.1mm)¡G\t0.000000\tVelocity(0.1mm0/s)¡G\t0.000000\tVoltage¡G\t0.005188\nReal Periold(ms)¡G\t1\tEncoder Position(0.1mm)¡G\t0.000000\tVelocity(0.1mm0/s)¡G\t0.000000\tVoltage¡G\t0.000427\nReal Periold(ms)¡G\t1\tEncoder Position(0.1mm)¡G\t0.000000\tVelocity(0.1mm0/s)¡G\t0.000000\tVoltage¡G\t-0.006592\nReal Periold(ms)¡G\t1\tEncoder Position(0.1mm)¡G\t0.000000\tVelocity(0.1mm0/s)¡G\t0.000000\tVoltage¡G\t0.004242\nReal Periold(ms)¡G\t1\tEncoder Position(0.1mm)¡G\t0.000000\tVelocity(0.1mm0/s)¡G\t0.000000\tVoltage¡G\t0.004547\nReal Periold(ms)¡G\t1\tEncoder Position(0.1mm)¡G\t0.000000\tVelocity(0.1mm0/s)¡G\t0.000000\tVoltage¡G\t0.000427\nReal Periold(ms)¡G\t1\tEncoder Position(0.1mm)¡G\t0.000000\tVelocity(0.1mm0/s)¡G\t0.000000\tVoltage¡G\t-0.006897\nReal Periold(ms)¡G\t1\tEncoder Position(0.1mm)¡G\t0.000000\tVelocity(0.1mm0/s)¡G\t0.000000\tVoltage¡G\t-0.006592\nReal Periold(ms)¡G\t1\tEncoder Position(0.1mm)¡G\t0.000000\tVelocity(0.1mm0/s)¡G\t0.000000\tVoltage¡G\t-0.004669\nReal Periold(ms)¡G\t1\tEncoder Position(0.1mm)¡G\t0.000000\tVelocity(0.1mm0/s)¡G\t0.000000\tVoltage¡G\t0.005524\nReal Periold(ms)¡G\t1\tEncoder Position(0.1mm)¡G\t0.000000\tVelocity(0.1mm0/s)¡G\t0.000000\tVoltage¡G\t-0.009125\nReal Periold(ms)¡G\t1\tEncoder Position(0.1mm)¡G\t0.000000\tVelocity(0.1mm0/s)¡G\t0.000000\tVoltage¡G\t0.004883\nReal Periold(ms)¡G\t1\tEncoder Position(0.1mm)¡G\t0.000000\tVelocity(0.1mm0/s)¡G\t0.000000\tVoltage¡G\t0.004883\nReal Periold(ms)¡G\t1\tEncoder Position(0.1mm)¡G\t0.000000\tVelocity(0.1mm0/s)¡G\t0.000000\tVoltage¡G\t0.000427\nReal Periold(ms)¡G\t1\tEncoder Position(0.1mm)¡G\t0.000000\tVelocity(0.1mm0/s)¡G\t0.000000\tVoltage¡G\t0.000092\nReal Periold(ms)¡G\t1\tEncoder Position(0.1mm)¡G\t0.000000\tVelocity(0.1mm0/s)¡G\t0.000000\tVoltage¡G\t-0.003723\nReal Periold(ms)¡G\t1\tEncoder Position(0.1mm)¡G\t0.000000\tVelocity(0.1mm0/s)¡G\t0.000000\tVoltage¡G\t0.000092\nReal Periold(ms)¡G\t1\tEncoder Position(0.1mm)¡G\t0.000000\tVelocity(0.1mm0/s)¡G\t0.000000\tVoltage¡G\t-0.008484\nReal Periold(ms)¡G\t1\tEncoder Position(0.1mm)¡G\t0.000000\tVelocity(0.1mm0/s)¡G\t0.000000\tVoltage¡G\t0.001373\nReal Periold(ms)¡G\t1\tEncoder Position(0.1mm)¡G\t0.000000\tVelocity(0.1mm0/s)¡G\t0.000000\tVoltage¡G\t0.006470\nReal Periold(ms)¡G\t1\tEncoder Position(0.1mm)¡G\t0.000000\tVelocity(0.1mm0/s)¡G\t0.000000\tVoltage¡G\t-0.003387\nReal Periold(ms)¡G\t1\tEncoder Position(0.1mm)¡G\t0.000000\tVelocity(0.1mm0/s)¡G\t0.000000\tVoltage¡G\t0.007751\nReal Periold(ms)¡G\t1\tEncoder Position(0.1mm)¡G\t0.000000\tVelocity(0.1mm0/s)¡G\t0.000000\tVoltage¡G\t-0.008179\nReal Periold(ms)¡G\t1\tEncoder Position(0.1mm)¡G\t0.000000\tVelocity(0.1mm0/s)¡G\t0.000000\tVoltage¡G\t-0.006256\nReal Periold(ms)¡G\t1\tEncoder Position(0.1mm)¡G\t0.000000\tVelocity(0.1mm0/s)¡G\t0.000000\tVoltage¡G\t-0.001160\nReal Periold(ms)¡G\t1\tEncoder Position(0.1mm)¡G\t0.000000\tVelocity(0.1mm0/s)¡G\t0.000000\tVoltage¡G\t0.003296\nReal Periold(ms)¡G\t1\tEncoder Position(0.1mm)¡G\t0.000000\tVelocity(0.1mm0/s)¡G\t0.000000\tVoltage¡G\t-0.001801\nReal Periold(ms)¡G\t1\tEncoder Position(0.1mm)¡G\t0.000000\tVelocity(0.1mm0/s)¡G\t0.000000\tVoltage¡G\t-0.004669\nReal Periold(ms)¡G\t1\tEncoder Position(0.1mm)¡G\t0.000000\tVelocity(0.1mm0/s)¡G\t0.000000\tVoltage¡G\t0.002960\nReal Periold(ms)¡G\t1\tEncoder Position(0.1mm)¡G\t0.000000\tVelocity(0.1mm0/s)¡G\t0.000000\tVoltage¡G\t0.000427\nReal Periold(ms)¡G\t1\tEncoder Position(0.1mm)¡G\t0.000000\tVelocity(0.1mm0/s)¡G\t0.000000\tVoltage¡G\t-0.015808\nReal Periold(ms)¡G\t1\tEncoder Position(0.1mm)¡G\t0.000000\tVelocity(0.1mm0/s)¡G\t0.000000\tVoltage¡G\t-0.003082\nReal Periold(ms)¡G\t1\tEncoder Position(0.1mm)¡G\t0.000000\tVelocity(0.1mm0/s)¡G\t0.000000\tVoltage¡G\t0.000732\nReal Periold(ms)¡G\t1\tEncoder Position(0.1mm)¡G\t0.000000\tVelocity(0.1mm0/s)¡G\t0.000000\tVoltage¡G\t0.000092\nReal Periold(ms)¡G\t1\tEncoder Position(0.1mm)¡G\t0.000000\tVelocity(0.1mm0/s)¡G\t0.000000\tVoltage¡G\t0.004883\nReal Periold(ms)¡G\t1\tEncoder Position(0.1mm)¡G\t0.000000\tVelocity(0.1mm0/s)¡G\t0.000000\tVoltage¡G\t0.000732\nReal Periold(ms)¡G\t1\tEncoder Position(0.1mm)¡G\t0.000000\tVelocity(0.1mm0/s)¡G\t0.000000\tVoltage¡G\t-0.004364\nReal Periold(ms)¡G\t1\tEncoder Position(0.1mm)¡G\t0.000000\tVelocity(0.1mm0/s)¡G\t0.000000\tVoltage¡G\t0.000427\nReal Periold(ms)¡G\t1\tEncoder Position(0.1mm)¡G\t0.000000\tVelocity(0.1mm0/s)¡G\t0.000000\tVoltage¡G\t0.001068\nReal Periold(ms)¡G\t1\tEncoder Position(0.1mm)¡G\t0.000000\tVelocity(0.1mm0/s)¡G\t0.000000\tVoltage¡G\t0.002319\nReal Periold(ms)¡G\t1\tEncoder Position(0.1mm)¡G\t0.000000\tVelocity(0.1mm0/s)¡G\t0.000000\tVoltage¡G\t-0.001495\nReal Periold(ms)¡G\t1\tEncoder Position(0.1mm)¡G\t0.000000\tVelocity(0.1mm0/s)¡G\t0.000000\tVoltage¡G\t0.009644\nReal Periold(ms)¡G\t1\tEncoder Position(0.1mm)¡G\t0.000000\tVelocity(0.1mm0/s)¡G\t0.000000\tVoltage¡G\t0.001373\nReal Periold(ms)¡G\t1\tEncoder Position(0.1mm)¡G\t0.000000\tVelocity(0.1mm0/s)¡G\t0.000000\tVoltage¡G\t-0.002136\nReal Periold(ms)¡G\t1\tEncoder Position(0.1mm)¡G\t0.000000\tVelocity(0.1mm0/s)¡G\t0.000000\tVoltage¡G\t-0.013916\nReal Periold(ms)¡G\t1\tEncoder Position(0.1mm)¡G\t0.000000\tVelocity(0.1mm0/s)¡G\t0.000000\tVoltage¡G\t0.002655\nReal Periold(ms)¡G\t1\tEncoder Position(0.1mm)¡G\t0.000000\tVelocity(0.1mm0/s)¡G\t0.000000\tVoltage¡G\t0.000427\nReal Periold(ms)¡G\t1\tEncoder Position(0.1mm)¡G\t0.000000\tVelocity(0.1mm0/s)¡G\t0.000000\tVoltage¡G\t0.000092\nReal Periold(ms)¡G\t1\tEncoder Position(0.1mm)¡G\t0.000000\tVelocity(0.1mm0/s)¡G\t0.000000\tVoltage¡G\t0.005524\nReal Periold(ms)¡G\t1\tEncoder Position(0.1mm)¡G\t0.000000\tVelocity(0.1mm0/s)¡G\t0.000000\tVoltage¡G\t-0.002441\nReal Periold(ms)¡G\t1\tEncoder Position(0.1mm)¡G\t0.000000\tVelocity(0.1mm0/s)¡G\t0.000000\tVoltage¡G\t-0.004364\nReal Periold(ms)¡G\t1\tEncoder Position(0.1mm)¡G\t0.000000\tVelocity(0.1mm0/s)¡G\t0.000000\tVoltage¡G\t-0.007843\nReal Periold(ms)¡G\t1\tEncoder Position(0.1mm)¡G\t0.000000\tVelocity(0.1mm0/s)¡G\t0.000000\tVoltage¡G\t-0.003082\nReal Periold(ms)¡G\t1\tEncoder Position(0.1mm)¡G\t0.000000\tVelocity(0.1mm0/s)¡G\t0.000000\tVoltage¡G\t0.013794\nReal Periold(ms)¡G\t1\tEncoder Position(0.1mm)¡G\t0.000000\tVelocity(0.1mm0/s)¡G\t0.000000\tVoltage¡G\t-0.018036\nReal Periold(ms)¡G\t1\tEncoder Position(0.1mm)¡G\t0.000000\tVelocity(0.1mm0/s)¡G\t0.000000\tVoltage¡G\t-0.008179\nReal Periold(ms)¡G\t1\tEncoder Position(0.1mm)¡G\t0.000000\tVelocity(0.1mm0/s)¡G\t0.000000\tVoltage¡G\t-0.017090\nReal Periold(ms)¡G\t1\tEncoder Position(0.1mm)¡G\t0.000000\tVelocity(0.1mm0/s)¡G\t0.000000\tVoltage¡G\t-0.009460\nReal Periold(ms)¡G\t1\tEncoder Position(0.1mm)¡G\t0.000000\tVelocity(0.1mm0/s)¡G\t0.000000\tVoltage¡G\t-0.000854\nReal Periold(ms)¡G\t1\tEncoder Position(0.1mm)¡G\t0.000000\tVelocity(0.1mm0/s)¡G\t0.000000\tVoltage¡G\t0.006134\nReal Periold(ms)¡G\t1\tEncoder Position(0.1mm)¡G\t0.000000\tVelocity(0.1mm0/s)¡G\t0.000000\tVoltage¡G\t-0.004669\nReal Periold(ms)¡G\t1\tEncoder Position(0.1mm)¡G\t0.000000\tVelocity(0.1mm0/s)¡G\t0.000000\tVoltage¡G\t-0.022827\nReal Periold(ms)¡G\t1\tEncoder Position(0.1mm)¡G\t0.000000\tVelocity(0.1mm0/s)¡G\t0.000000\tVoltage¡G\t-0.004669\nReal Periold(ms)¡G\t1\tEncoder Position(0.1mm)¡G\t0.000000\tVelocity(0.1mm0/s)¡G\t0.000000\tVoltage¡G\t0.003296\nReal Periold(ms)¡G\t1\tEncoder Position(0.1mm)¡G\t0.000000\tVelocity(0.1mm0/s)¡G\t0.000000\tVoltage¡G\t0.016327\nReal Periold(ms)¡G\t1\tEncoder Position(0.1mm)¡G\t0.000000\tVelocity(0.1mm0/s)¡G\t0.000000\tVoltage¡G\t0.048157\nReal Periold(ms)¡G\t1\tEncoder Position(0.1mm)¡G\t0.000000\tVelocity(0.1mm0/s)¡G\t0.000000\tVoltage¡G\t-0.005615\nReal Periold(ms)¡G\t1\tEncoder Position(0.1mm)¡G\t0.000000\tVelocity(0.1mm0/s)¡G\t0.000000\tVoltage¡G\t0.001678\nReal Periold(ms)¡G\t1\tEncoder Position(0.1mm)¡G\t0.000000\tVelocity(0.1mm0/s)¡G\t0.000000\tVoltage¡G\t0.009644\nReal Periold(ms)¡G\t1\tEncoder Position(0.1mm)¡G\t0.000000\tVelocity(0.1mm0/s)¡G\t0.000000\tVoltage¡G\t0.003601\nReal Periold(ms)¡G\t1\tEncoder Position(0.1mm)¡G\t0.000000\tVelocity(0.1mm0/s)¡G\t0.000000\tVoltage¡G\t-0.011688\nReal Periold(ms)¡G\t1\tEncoder Position(0.1mm)¡G\t0.000000\tVelocity(0.1mm0/s)¡G\t0.000000\tVoltage¡G\t-0.012299\nReal Periold(ms)¡G\t1\tEncoder Position(0.1mm)¡G\t0.000000\tVelocity(0.1mm0/s)¡G\t0.000000\tVoltage¡G\t0.002655\nReal Periold(ms)¡G\t1\tEncoder Position(0.1mm)¡G\t0.000000\tVelocity(0.1mm0/s)¡G\t0.000000\tVoltage¡G\t-0.014221\nReal Periold(ms)¡G\t1\tEncoder Position(0.1mm)¡G\t0.000000\tVelocity(0.1mm0/s)¡G\t0.000000\tVoltage¡G\t0.002655\nReal Periold(ms)¡G\t1\tEncoder Position(0.1mm)¡G\t0.000000\tVelocity(0.1mm0/s)¡G\t0.000000\tVoltage¡G\t0.006775\nReal Periold(ms)¡G\t1\tEncoder Position(0.1mm)¡G\t0.000000\tVelocity(0.1mm0/s)¡G\t0.000000\tVoltage¡G\t0.000732\nReal Periold(ms)¡G\t1\tEncoder Position(0.1mm)¡G\t0.000000\tVelocity(0.1mm0/s)¡G\t0.000000\tVoltage¡G\t-0.005310\nReal Periold(ms)¡G\t1\tEncoder Position(0.1mm)¡G\t0.000000\tVelocity(0.1mm0/s)¡G\t0.000000\tVoltage¡G\t0.004547\nReal Periold(ms)¡G\t1\tEncoder Position(0.1mm)¡G\t0.000000\tVelocity(0.1mm0/s)¡G\t0.000000\tVoltage¡G\t-0.004669\nReal Periold(ms)¡G\t1\tEncoder Position(0.1mm)¡G\t0.000000\tVelocity(0.1mm0/s)¡G\t0.000000\tVoltage¡G\t-0.002777\nReal Periold(ms)¡G\t1\tEncoder Position(0.1mm)¡G\t0.000000\tVelocity(0.1mm0/s)¡G\t0.000000\tVoltage¡G\t0.002014\nReal Periold(ms)¡G\t1\tEncoder Position(0.1mm)¡G\t0.000000\tVelocity(0.1mm0/s)¡G\t0.000000\tVoltage¡G\t0.001373\nReal Periold(ms)¡G\t1\tEncoder Position(0.1mm)¡G\t0.000000\tVelocity(0.1mm0/s)¡G\t0.000000\tVoltage¡G\t0.000732\nReal Periold(ms)¡G\t1\tEncoder Position(0.1mm)¡G\t0.000000\tVelocity(0.1mm0/s)¡G\t0.000000\tVoltage¡G\t0.007751\nReal Periold(ms)¡G\t1\tEncoder Position(0.1mm)¡G\t0.000000\tVelocity(0.1mm0/s)¡G\t0.000000\tVoltage¡G\t-0.005005\nReal Periold(ms)¡G\t1\tEncoder Position(0.1mm)¡G\t0.000000\tVelocity(0.1mm0/s)¡G\t0.000000\tVoltage¡G\t-0.012299\nReal Periold(ms)¡G\t1\tEncoder Position(0.1mm)¡G\t0.000000\tVelocity(0.1mm0/s)¡G\t0.000000\tVoltage¡G\t
